vi "Acknowledge.vi"(8 "error in (no error)":errorcluster) -> (0 "error out":errorcluster)   [LabVIEW 2021, in "Error Handler Actor API.lvclass"]
uses:
  Error Handler Actor API.lvclass
  Re-use Libraries/Minimal Actor Framework/Messaging/Message/Message.lvclass
  Error Handler Actor API.lvclass/Error Handler Actor API.ctl
  Globals.vi
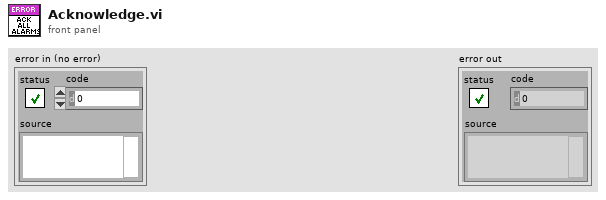
[diagram p1: front panel]
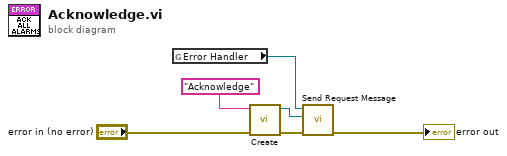
[diagram p0: block diagram]
diagram:
  n1 = global read "Globals.vi" "Error Handler"() -> (w1:refnum<class "Error Handler Actor API.lvclass">)
  n2 = call "Create.vi"("error in (no error)"="error in (no error)", "Name"="Acknowledge" ("Parameter")) -> ("error out"=w2:errorcluster, "Message out"=w3:refnum<class "Message.lvclass">)  [unwired: 8 in]
  n3 = call-dynamic "Send Request Message.vi"("error in (no error)"=w2, "Message"=w3, "Actor API in"=w1) -> ("error out"=→"error out":errorcluster)  [unwired: 8 in]
